vi "MSScript_SubVI_SortBlockComment.vi"(1 "RecoverySEL input":cluster{"Start":u32, "End":u32}[](array[cluster])) -> (0 "RecoverySEL output":cluster{"Start":u32, "End":u32}[](array[cluster]))   [LabVIEW 2018, in "MSScript.lvclass"]
uses:
  MSScript.lvclass
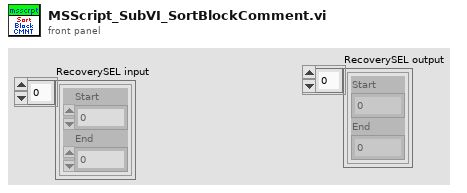
[diagram p1: front panel]
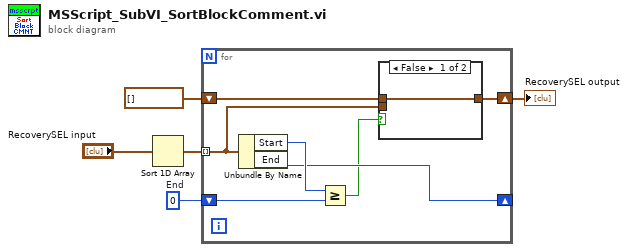
[diagram p0: block diagram]
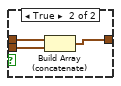
[diagram p2: hidden frame]
diagram:
  w2 = u32 0  # End
  n1 = Sort 1D Array(array="RecoverySEL input") -> (sorted array=w4:cluster{"Start":u32, "End":u32}[])
  n2 = for {
    tunnel: w4 -> [w7] mode=indexing
    shift-right: [w6] -> w1
    shift-left: cluster{"Start":u32, "End":u32}[] [] ("RecoverySEL") -> [w8]
    shift-right: [w10] -> _
    shift-left: w2 -> [w11]
    n3 = Unbundle By Name(w7) -> ("Start"=w12:u32, "End"=w10:u32)
    n4 = Greater Or Equal?(x=w12, y=w11) -> (x >= y?=w9:bool)
    n5 = case shown="False" w9 {
      tunnel: w8 -> [w13 w16]
      tunnel: w7 -> [_ w15]
      tunnel: [w13 w14] -> w6
      frame False {
      }
      frame True {
        n6 = Build Array (concatenate)(w16, w15) -> (w14:cluster{"Start":u32, "End":u32}[])
      }
    }
  }
  "RecoverySEL output" <- w1
